vi "Expt7_MT MSK Transceiver_Student_lab.vi"(0 "# Message Symbols":i32=1000, 7 "Eb/N0, dB":dbl(slide)=40.0 scale=0.0..80.0, 11 "Reset":bool=TRUE, 14 "?":T2(tab)=enum."MSK Constellation (RX)") -> (3 "MSK System Parameters":T5={"Differential Encoding Enable"=enum."enable", "Samples per Symbol (16)"=16}, 4 "Output Complex Waveform":cluster{"t0":dbl, "dt":dbl, "Values":cdb[]} {"Values" format="%.3f"; "dt" format="%^.2e"; "t0" format="%.4f"}, 6 "Transmitted Bits":i8[](array[numeric]), 8 "Received  Bits":i8[](array[numeric]), 10 "Bit Error Rate":dbl format="%.4e", 13 "Last Sync Found Index":dbl format="%.4f", 15 "Error Out":errorcluster)   [LabVIEW 2020]
doc: "This example demonstrates generation and analysis of MSK modulated signals. You can specify transmit filter parameters, Eb/No, and frequency offset. This example demonstrates programming techniques for resetting the transmitter in cases where the receiver (demodulator) lock is lost. You can see the results of the demodulation on trellis graphs, and perform measurements such as bit error rate."
uses:
  <vilib>/addons/Modulation/niDMT.lvlib
panel:
  out "Estimated Eb/N0(dB)":dbl
  out "Sampling Rate":dbl format="%.2p"
  in  "BT":dbl=0.5 format="%.2f"
  out "Frequency Offset (Hz)":dbl format="%.2f"
  in  "Frequency Offset (Hz)":dbl(slide) scale=-1000.0..1000.0
  in  "Symbol Rate":dbl=100000.0 step=1000.0 format="%.2p"
  out "Modulation Error Ratio (dB)":dbl format="%.2f"
  out "BER Trigger Found ?":bool
  in  "TX Filter":T1(ring)=enum."Gaussian"
  in  "?":bool
  out "TX Symbols":T3(graph)={{"1/x"=0.0, 1e-05, [], 1}, []}
  out "TX Constellation":T4(graph)
  out "TX Trellis graph":cluster{dbl, "dt":dbl, dbl[]}[](graph)
  out "RX Symbols":T3(graph)={{"1/x"=0.0, 1e-05, [], 1}, []}
  in  "autoscale":bool
  out "RX Constellation":T4(graph)
  out "RX Trellis Graph":cluster{dbl, "dt":dbl, dbl[]}[](graph)
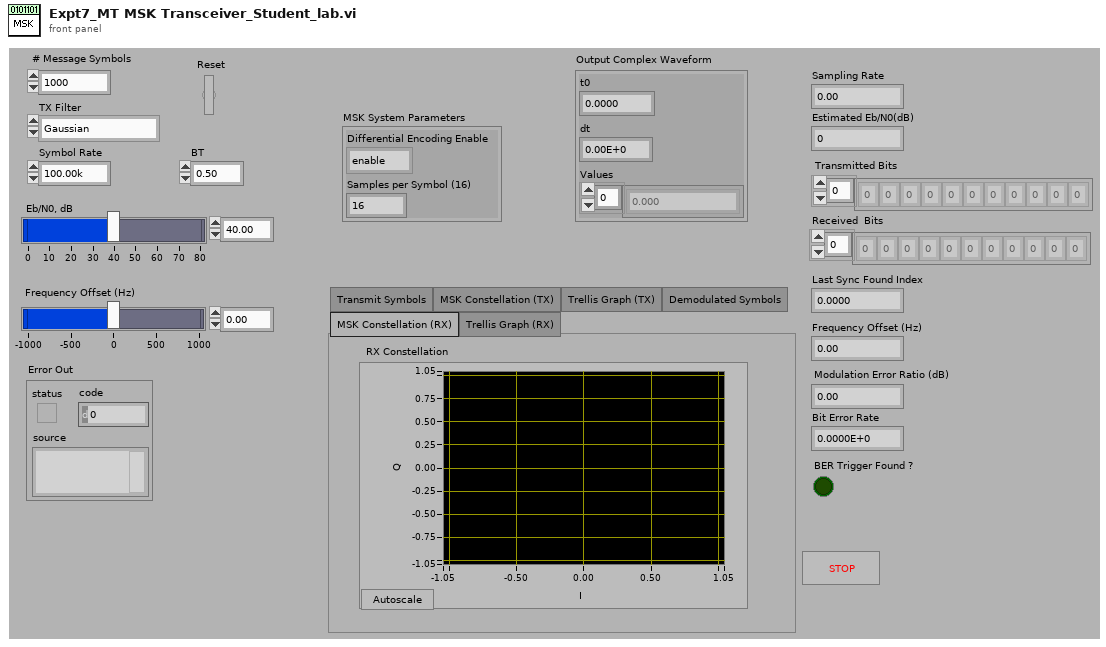
[diagram p1: front panel]
types:
  T1 = enum16{"none", "Raised Cosine", "Root Raised Cos", "Gaussian"}
  T2 = enum32{"Transmit Symbols", "MSK Constellation (TX)", "Trellis Graph (TX)", "Demodulated Symbols", "MSK Constellation (RX)", "Trellis Graph (RX)"}
  T3 = cluster{cluster{"1/x":dbl, dbl, i8[], i32}, i32[][]}
  T4 = cluster{"Decimated Array":dbl[], "Decimated Array":dbl[]}[]
  T5 = cluster{"Differential Encoding Enable":enum16{"disable", "enable"}, "Samples per Symbol (16)":i32}
  T6 = cluster{"expected sync location (symbols)":i32, "sync sequence":cdb[], "sync location uncertainty (symbols)":i32, "sync indent (symbols)":i32}
  T7 = cluster{"TX Filter":enum16{"none", "Raised Cosine", "Root Raised Cos", "Gaussian"}, "filter parameter":dbl, "filter length":i32}
  T8 = cluster{"# Guard Bits":i32, "# Sync Bits":i32, "# Message Bits":i32, "PN sequence order":i32}
  T9 = cluster{"constellation":dbl[], "oversampled data":dbl[]}[]
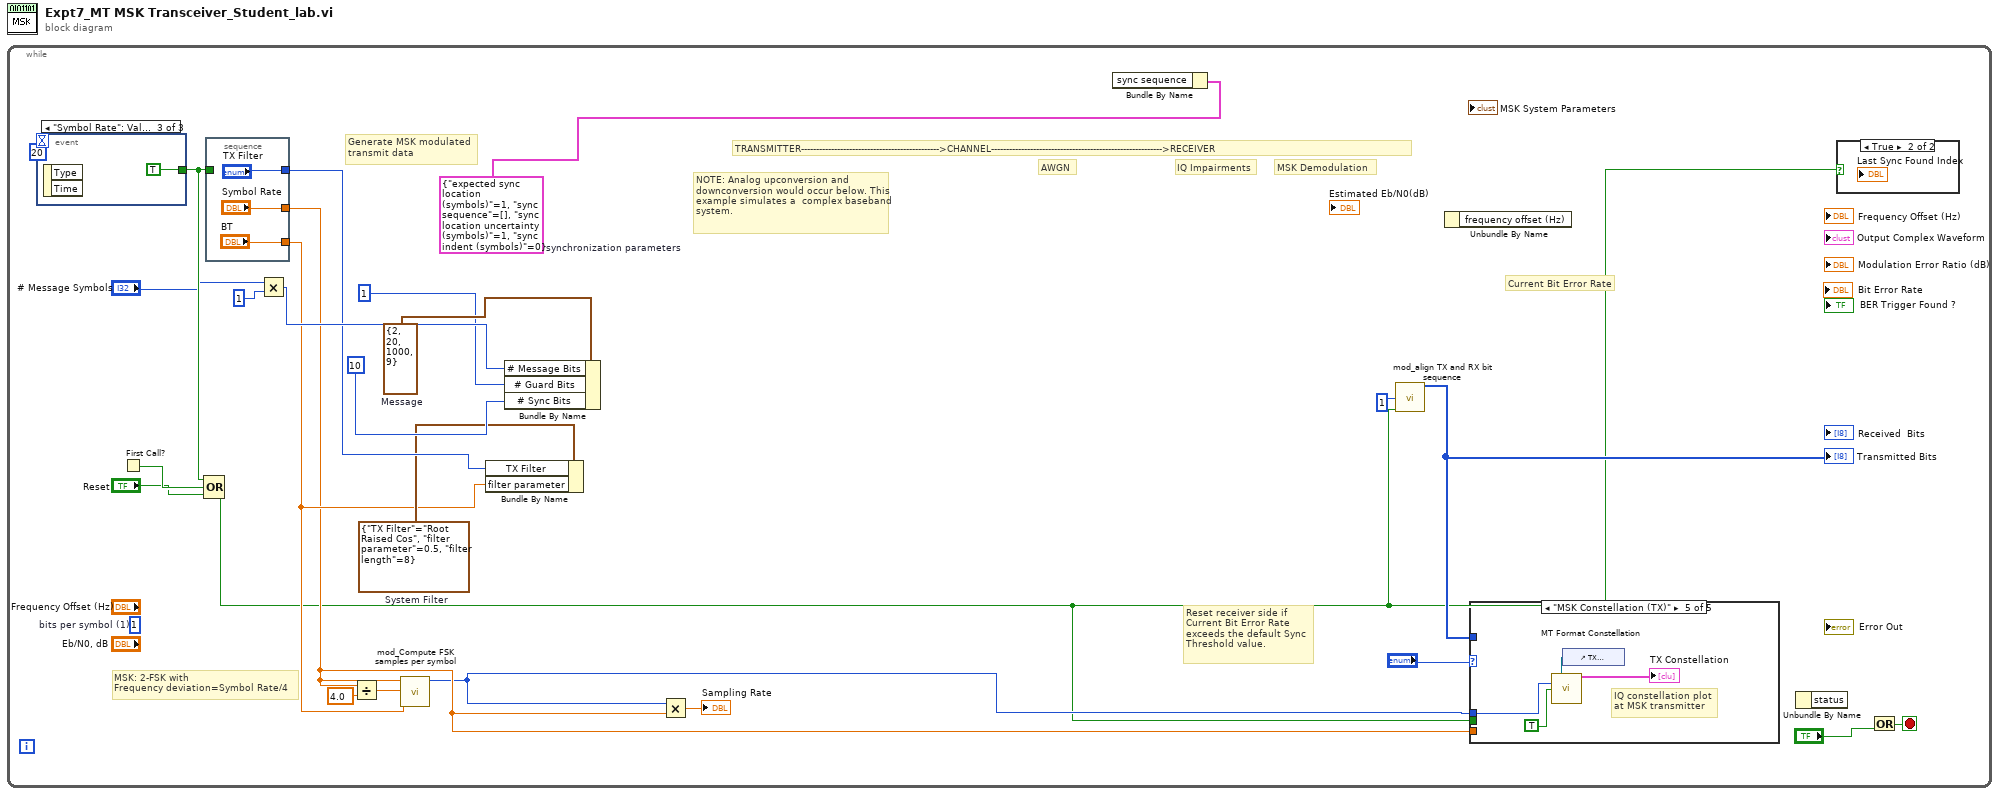
[diagram p0: block diagram]
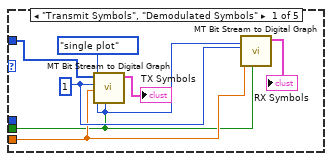
[diagram p2: hidden frame]
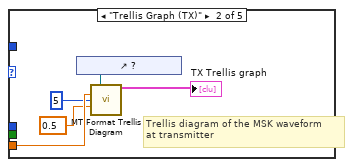
[diagram p3: hidden frame]
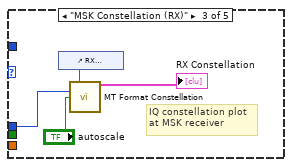
[diagram p4: hidden frame]
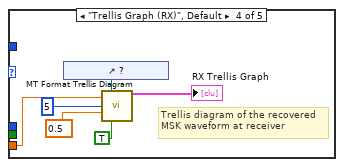
[diagram p5: hidden frame]
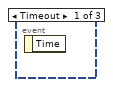
[diagram p7: hidden frame]
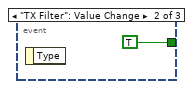
[diagram p8: hidden frame]
diagram:
  n1 = while {
    stop <- w13 stop-if-true
    w3 = T6 {"expected sync location (symbols)"=1, "sync sequence"=[], "sync location uncertainty (symbols)"=1, "sync indent (symbols)"=0}  # synchronization parameters
    w10 = T7 {"TX Filter"=enum."Root Raised Cos", "filter parameter"=0.5, "filter length"=8}  # System Filter
    (unwired) 1  # bits per symbol (1)
    w19 = T8 {"# Guard Bits"=2, "# Sync Bits"=20, "# Message Bits"=1000, "PN sequence order"=9}  # Message
    # "IQ Impairments"
    # "NOTE: Analog upconversion and downconversion would occur below. This example simulates a  complex baseband system."
    # "MSK: 2-FSK with\nFrequency deviation=Symbol Rate/4"
    # "Reset receiver side if \nCurrent Bit Error Rate\nexceeds the default Sync \nThreshold value."
    # "AWGN"
    # "Generate MSK modulated\ntransmit data"
    # "MSK Demodulation"
    # "Current Bit Error Rate"
    # "TRANSMITTER---------------------------------------------->CHANNEL--------------------------------------------------------->RECEIVER"
    n2 = event shown="[2] \"Symbol Rate\": Value Change" {
      selector: _ -> [_ _ _]
      dyn-events: _ -> [_ _ _]
      timeout: 20 -> [_ _ _]
      tunnel: [_ TRUE TRUE] -> w21
      event Timeout {
        n3 = event-data() -> ()  [unwired: 1 in, 1 out]
      }
      event "TX Filter": Value Change {
        n4 = event-data() -> ()  [unwired: 1 in, 1 out]
      }
      event "Symbol Rate": Value Change {
        n5 = event-data() -> ()  [unwired: 1 in, 2 out]
      }
    }
    n6 = First Call?() -> (First Call?: T/F=w24:bool)
    n7 = Compound Arithmetic op=OR(w21, w24, "Reset") -> (w1:bool)
    n8 = stacked-sequence {
      tunnel: w21 -> [_]
      tunnel: ["TX Filter"] -> w16
      tunnel: ["Symbol Rate"] -> w5
      tunnel: ["BT"] -> w6
      frame #0 {
      }
    }
    n9 = Multiply(x="# Message Symbols", y=1) -> (x*y=w17:i32)
    n10 = Divide(x=w5, y=4.0) -> (x/y=w8:dbl)
    n11 = call <vilib>:"mod_Compute FSK samples per symbol.vi"("Symbol Rate"=w5, "Deviation (Hz)"=w8, "Filter parameter"=w6) -> ("FSK samples per symbol"=w2:i32)  [unwired: 11 in, 1 out]
    n12 = Bundle By Name(cluster=w10, "TX Filter"=w16, "filter parameter"=w6) -> ()  [unwired: 1 out]
    n13 = Bundle By Name(cluster=w19, "# Message Bits"=w17, "# Guard Bits"=1, "# Sync Bits"=10) -> ()  [unwired: 1 out]
    n14 = Multiply(x=w2, y=w5) -> (x*y=→"Sampling Rate":dbl)
    n15 = Bundle By Name(cluster=w3) -> ()  [unwired: 1 in, 1 out]
    n16 = call <vilib>:"mod_align TX and RX bit sequence.vi"("# Bits removed"=1, "Reset"=w1) -> ("Aligned array"=w14:i8[])  [unwired: 13 in]
    "Transmitted Bits" <- w14
    n17 = Unbundle By Name() -> ()  [unwired: 1 in, 1 out]
    n18 = case shown="\"MSK Constellation (TX)\"" "?" {
      tunnel: w5 -> [w33 w38 _ w48 _]
      tunnel: w2 -> [_ _ w42 _ w51]
      tunnel: w14 -> [w30 _ _ _ _]
      tunnel: w1 -> [w31 _ _ _ _]
      frame "Transmit Symbols", "Demodulated Symbols" {
        w32 = enum16{"single plot", "plot per bit"}."single plot" ("Format")
        w34 = 1 ("bits per symbol")
        n19 = call <vilib>:"MT Bit Stream to Digital Graph.vi"("Reset (F)"=w31, "Format"=w32, "Symbol Rate (Hz)"=w33, "bits per symbol"=w34, "Bit Stream"=w30) -> ("Digital Waveform Graph"=→"TX Symbols":T3)  [unwired: 6 in]
        n20 = call <vilib>:"MT Bit Stream to Digital Graph.vi"("Reset (F)"=w31, "Format"=w32, "Symbol Rate (Hz)"=w33, "bits per symbol"=w34) -> ("Digital Waveform Graph"=→"RX Symbols":T3)  [unwired: 7 in]
      }
      frame "Trellis Graph (TX)" {
        # "Trellis diagram of the MSK waveform \nat transmitter"
        n21 = control-ref of="?"() -> (w39:refnum<vi>)
        n22 = call <vilib>:"MT Format Trellis Diagram.vi"("trellis reference"=w39, "symbol rate (Hz)"=w38, "trellis length"=5, "modulation index"=0.5) -> ("trellis diagram"=→"TX Trellis graph":cluster{"t0":dbl, "dt":dbl, "phase":dbl[]}[])  [unwired: 10 in, 1 out]
      }
      frame "MSK Constellation (RX)" {
        # "IQ constellation plot\nat MSK receiver"
        n23 = control-ref of="RX Constellation"() -> (w43:refnum<vi>)
        n24 = call <vilib>:"MT Format Constellation.vi"("constellation reference"=w43, "samples per symbol"=w42, "autoscale"="autoscale") -> ("constellation graph"=→"RX Constellation":T9)  [unwired: 11 in, 1 out]
      }
      frame "Trellis Graph (RX)", Default {
        # "Trellis diagram of the recovered\nMSK waveform at receiver"
        n25 = control-ref of="?"() -> (w49:refnum<vi>)
        n26 = call <vilib>:"MT Format Trellis Diagram.vi"("trellis reference"=w49, "symbol rate (Hz)"=w48, "trellis length"=5, "modulation index"=0.5, "autoscale"=TRUE) -> ("trellis diagram"=→"RX Trellis Graph":cluster{"t0":dbl, "dt":dbl, "phase":dbl[]}[])  [unwired: 9 in, 1 out]
      }
      frame "MSK Constellation (TX)" {
        # "IQ constellation plot\nat MSK transmitter"
        n27 = control-ref of="TX Constellation"() -> (w53:refnum<vi>)
        n28 = call <vilib>:"MT Format Constellation.vi"("constellation reference"=w53, "samples per symbol"=w51, "autoscale"=TRUE) -> ("constellation graph"=→"TX Constellation":T9)  [unwired: 11 in, 1 out]
      }
    }
    n29 = Unbundle By Name() -> ()  [unwired: 1 in, 1 out]
    n30 = case shown="True" w1 {
      frame False {
      }
      frame True {
      }
    }
    n31 = Or(y="?") -> (x .or. y?=w13:bool)  [unwired: 1 in]
  }
